vi "Perform Action.vi"(8 "error in (no error)":errorcluster, 11 "ITask Actor in":refnum<class "ITask Actor.lvclass">) -> (0 "error out":errorcluster, 3 "ITask Actor out":refnum<class "ITask Actor.lvclass">)   [LabVIEW 2023, in "ITask Actor.lvlib" / "ITask Actor.lvclass"]
uses:
  ITask Actor.lvclass
  <vilib>/Utility/error.llb/Error Cluster From Error Code.vi
  <vilib>/ErrorRing/Error Ring.xnode
panel:
  out "Output":variant
  out "Input":variant
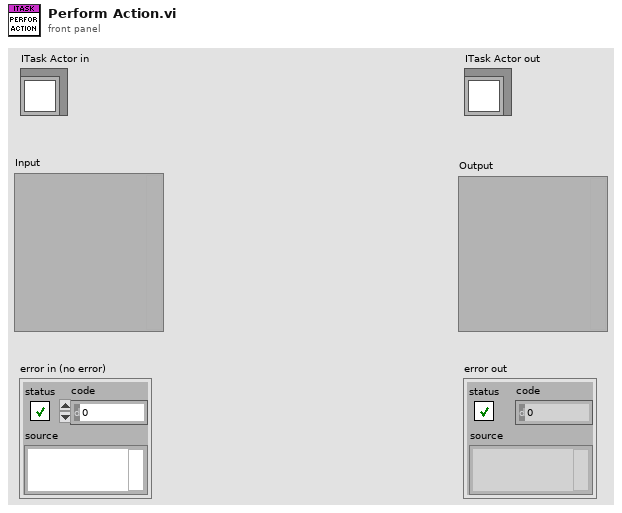
[diagram p1: front panel]
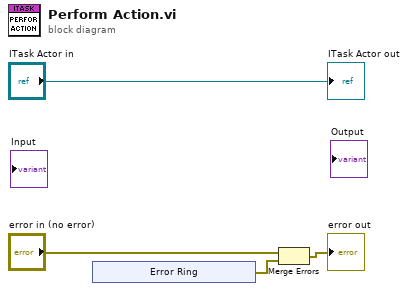
[diagram p0: block diagram]
diagram:
  n1 = xnode "Error Ring"() -> ("error out"=w1:errorcluster)
  n2 = Merge Errors("error in (no error)", w1) -> (→"error out":errorcluster)
  "ITask Actor out" <- "ITask Actor in"
